vi "Get Per-Site Ref Mic Senstivity.vi"(0 "TSM context":T1, 11 "error in (no error)":errorcluster) -> (4 "Per-Site Ref Mic Sensitivity (mV/Pa)":dbl[](array[numeric]), 6 "Found?":bool, 15 "error out":errorcluster)   [LabVIEW 2020]
doc: "Gets the Reference Mic Sensitivity (mV/Pa) for each site from the Reference Mic Calibration Data"
uses:
  <vilib>/NI_TestStand_SemiconductorModule/NI_TestStand_Semiconductor_Module.lvlibp/PinMap/General/SemiconductorModuleContext.ctl
  <vilib>/NI_TestStand_SemiconductorModule/NI_TestStand_Semiconductor_Module.lvlibp
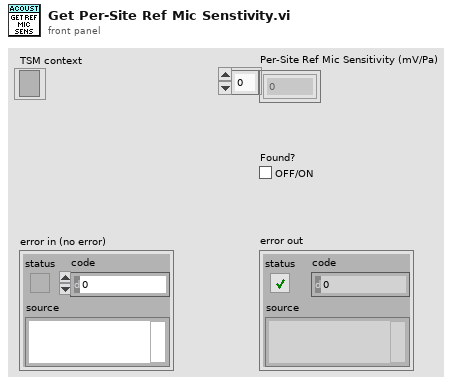
[diagram p1: front panel]
types:
  T1 = typedef "NI_TestStand_Semiconductor_Module.lvlibp/SemiconductorModuleContext.ctl" = refnum<k7>
  T2 = typedef "Acoustic Cal Data Cluster.ctl" = cluster{"Site Number":i32, "Serial Number":u32, "Ref Mic Sensitivity":dbl, "SPL Axis":dbl[], "Frequency Axis":dbl[], "Speaker Vp":dbl[][], "Ref Mic Cal File Data":string[][], "Speaker Vp Axis":dbl[], "SPL Measurements":dbl[][]}
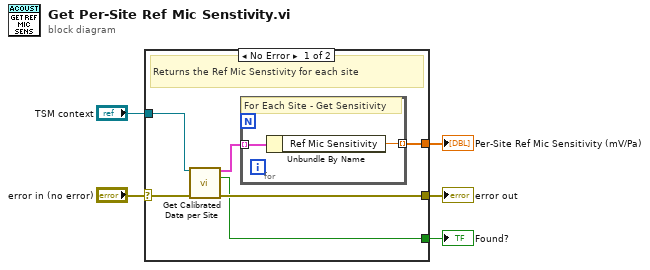
[diagram p0: block diagram]
diagram:
  n1 = case shown="No Error" "error in (no error)" {
    selector: "error in (no error)" -> [w10 w14]
    tunnel: "TSM context" -> [w11 _]
    tunnel: [w9 w14] -> w3
    tunnel: [w8 _] -> w2
    tunnel: [w6 _] -> w1
    frame No Error {
      # "Returns the Ref Mic Senstivity for each site"
      n2 = call "Get Calibrated Data per Site.vi"("TSM context"=w11, "error in (no error)"=w10) -> ("Per Site Acoustic Cal Data"=w7:T2[], "Found?"=w8:bool, "error out"=w9:errorcluster)  [unwired: 11 in]
      n3 = for {
        tunnel: w7 -> [w13] mode=indexing
        tunnel: [w12] -> w6 mode=indexing
        # "For Each Site - Get Sensitivity"
        n4 = Unbundle By Name(w13) -> ("Ref Mic Sensitivity"=w12:dbl)
      }
    }
    frame Error {
      # "Error - Do Nothing"
    }
  }
  "error out" <- w3
  "Found?" <- w2
  "Per-Site Ref Mic Sensitivity (mV/Pa)" <- w1
